vi "MAIN SINUS PENTA.vi"(8 "err in":errorcluster, 10 "SIMULAZIONE":bool=TRUE) -> ()   [LabVIEW 2019]
uses:
  controls/Parametri inverter letti.ctl
  controls/Dati targa sinus penta.ctl
  <vilib>/Utility/file.llb/Read Delimited Spreadsheet (string).vi
  Global dati targa SINUSPENTA.vi
  <vilib>/Modbus/master/Create Master Instance (Serial).vi
  <vilib>/Modbus/master/Modbus Master.lvclass
panel:
  out "register values":u16[](array[numeric])
  in  "modalità stop":i16
  in  "set modalità stop":bool
  out "error out":errorcluster
  out "appended array 3":u16[](array[numeric])
  out "appended array 2":dbl[](array[numeric])
  in  "DATI TARGA sinus penta 2":T1 {"Potenza nominale del motore Mot1" format="%.1f"; "Corrente nominale del motore Mot1" format="%.1f"; "Tensione nominale del motore mot1" format="%.1f"}
  out "# elements in queue":i32
  in  "START ABILITA":bool
  out "data 2":dbl
  out "Freq nominale del motore Mot1":u16
  out "DATI TARGA sinus penta":T1
  out "appended array":u16[](array[numeric])
  out "RPM nominali del motore Mot1":u16
  in  "set dati targa":bool
  in  "set rampa":bool
  in  "rampa":dbl
  in  "connetti":bool
  in  "disconnetti":bool
  out "data":dbl
  in  "Abilitato":bool
  in  "in marcia":bool=TRUE
  in  "SETUP PORTA SERIALE":T2={"Porta COM"="COM8", "Baud Rate"=38400, "Parity"=0, "Flow Control"=0, "Timeout"=10000, "Mode"=enum."RTU", "Slave Address"=1} {"Flow Control" items=["None", "XON/XOFF", "RTS/CTS", "XON/XOFF & RTS/CTS", "DTR/DSR", "XON/XOFF & DTR/DSR"]; "Parity" items=["None", "Odd", "Even", "Mark", "Space"]}
  out "t":errorcluster
  in  "Visualizza numero registri":bool
  in  "stop":bool
  in  "holding register values":i16[](array[numeric])
  in  "starting address":u16
  in  "write register":bool
  out "READ SINUS PENTA":T3
  out "Numeric":i32
  out "STATO":string
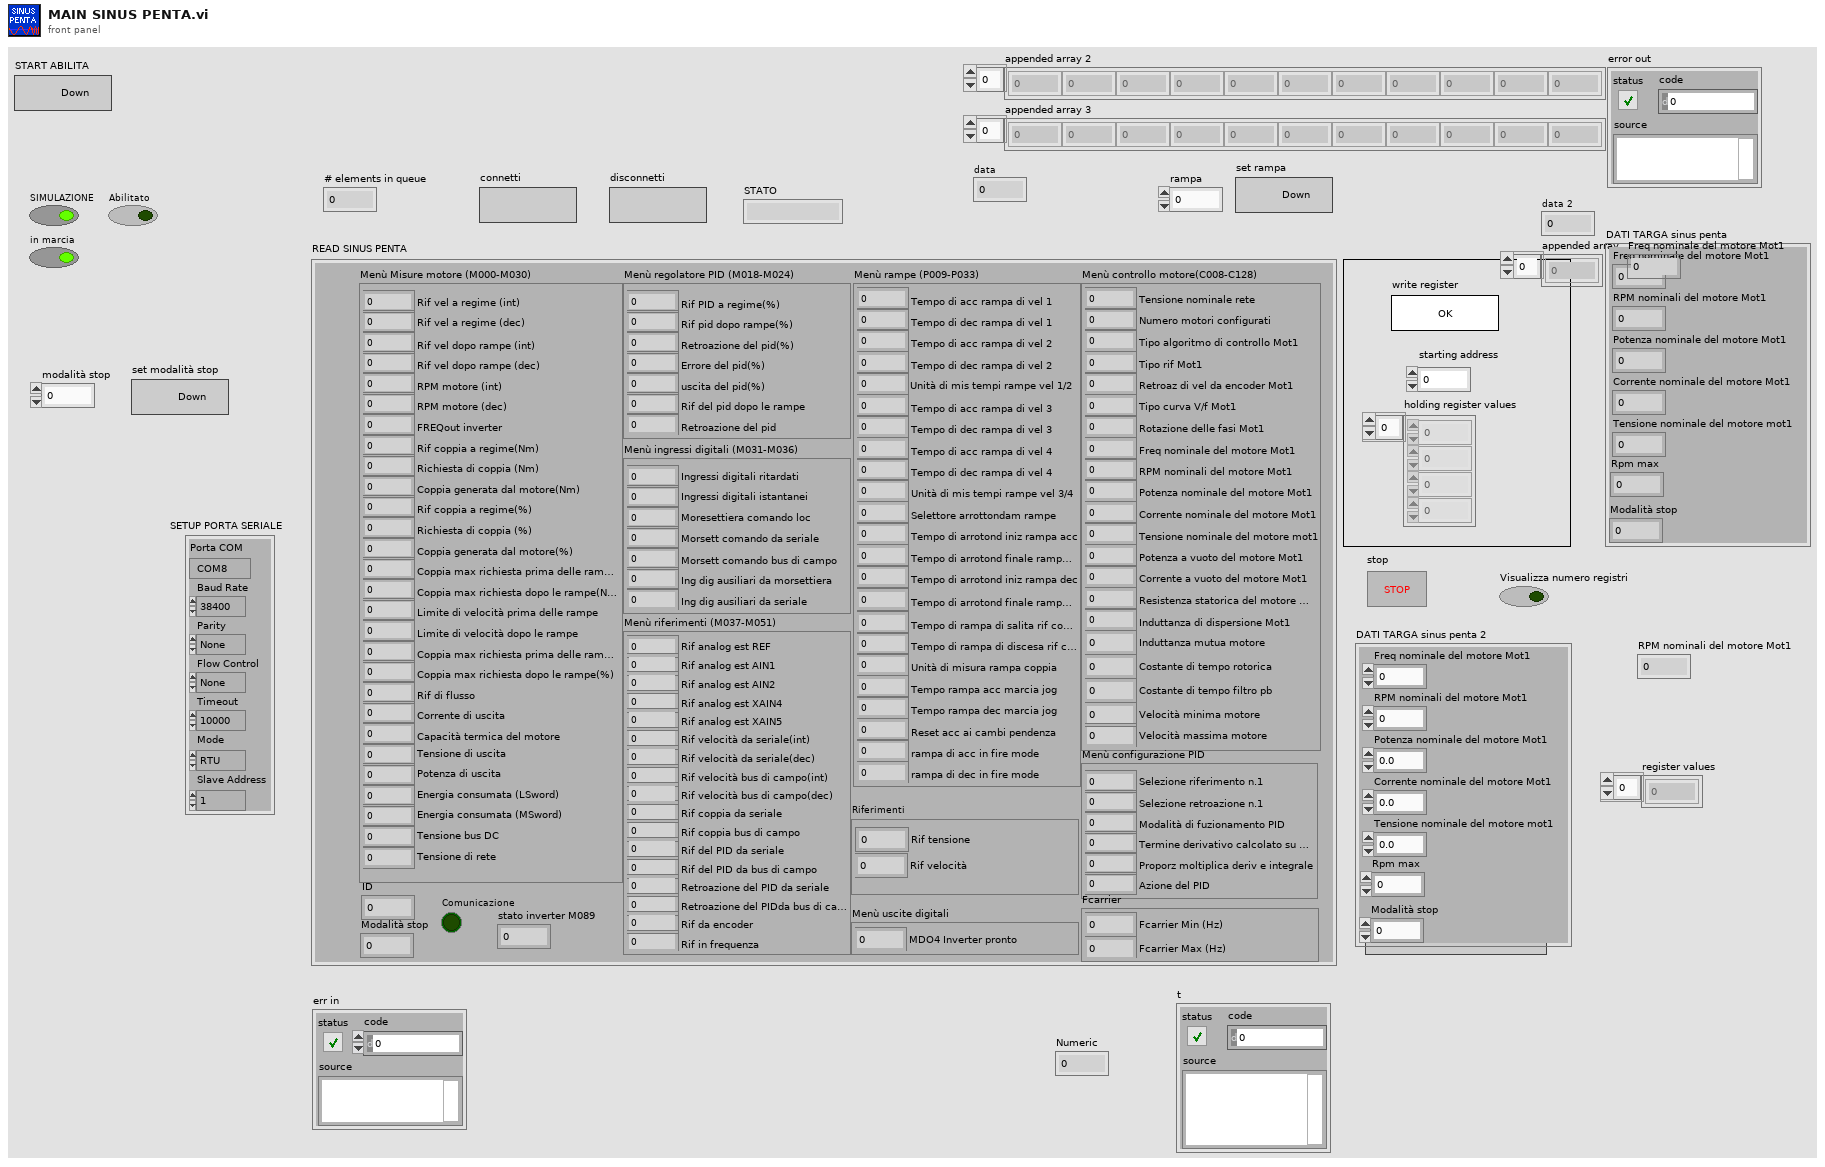
[diagram p1: front panel]
types:
  T1 = typedef "Dati targa sinus penta.ctl" = cluster{"Freq nominale del motore Mot1":dbl, "RPM nominali del motore Mot1":i16, "Potenza nominale del motore Mot1":dbl, "Corrente nominale del motore Mot1":dbl, "Tensione nominale del motore mot1":dbl, "Rpm max":u16, "Modalità stop":u16}
  T2 = cluster{"Porta COM":string, "Baud Rate":u32, "Parity":u16, "Flow Control":u16, "Timeout":u32, "Mode":enum16{"RTU", "ASCII"}, "Slave Address":u8}
  T3 = typedef "Parametri inverter letti.ctl" = cluster{"Menù Misure motore (M000-M030)":cluster{"Rif vel a regime (int)":u16, "Rif vel a regime (dec)":u16, "Rif vel dopo rampe (int)":u16, "Rif vel dopo rampe (dec)":u16, "RPM motore (int)":u16, "RPM motore (dec)":u16, "FREQout inverter":u16, "Rif coppia a regime(Nm)":u16, "Richiesta di coppia (Nm)":u16, "Coppia generata dal motore(Nm)":u16, "Rif coppia a regime(%)":u16, "Richiesta di coppia (%)":u16, "Coppia generata dal motore(%)":u16, "Coppia max richiesta prima delle rampe(Nm)":u16, "Coppia max richiesta dopo le rampe(Nm)":u16, "Limite di velocità prima delle rampe":u16, "Limite di velocità dopo le rampe":u16, "Coppia max richiesta prima delle rampe(%)":u16, "Coppia max richiesta dopo le rampe(%)":u16, "Rif di flusso":u16, "Corrente di uscita":u16, "Capacità termica del motore":u16, "Tensione di uscita":u16, "Potenza di uscita":u16, "Energia consumata (LSword)":u16, "Energia consumata (MSword)":u16, "Tensione bus DC":u16, "Tensione di rete":u16}, "Menù regolatore PID (M018-M024)":cluster{"Rif PID a regime(%)":u16, "Rif pid dopo rampe(%)":u16, "Retroazione del pid(%)":u16, "Errore del pid(%)":u16, "uscita del pid(%)":u16, "Rif del pid dopo le rampe":u16, "Retroazione del pid":u16}, "Menù ingressi digitali (M031-M036)":cluster{"Ingressi digitali ritardati":u16, "Ingressi digitali istantanei":u16, "Moresettiera comando loc":u16, "Morsett comando da seriale":u16, "Morsett comando bus di campo":u16, "Ing dig ausiliari da morsettiera":u16, "Ing dig ausiliari da seriale":u16}, "Menù riferimenti (M037-M051)":cluster{"Rif analog est REF":u16, "Rif analog est AIN1":u16, "Rif analog est AIN2":u16, "Rif analog est XAIN4":u16, "Rif analog est XAIN5":u16, "Rif velocità da seriale(int)":u16, "Rif velocità bus di campo(int)":u16, "Rif coppia da seriale":u16, "Rif coppia bus di campo":u16, "Rif del PID da seriale":u16, "Rif del PID da bus di campo":u16, "Retroazione del PID da seriale":u16, "Retroazione del PIDda bus di campo":u16, "Rif da encoder":u16, "Rif in frequenza":u16, "Rif velocità da seriale(dec)":u16, "Rif velocità bus di campo(dec)":u16}, "Menù rampe (P009-P033)":cluster{"Tempo di dec rampa di vel 1":u16, "Tempo di acc rampa di vel 2":u16, "Tempo di dec rampa di vel 2":u16, "Tempo di acc rampa di vel 1":u16, "Unità di mis tempi rampe vel 1/2":u16, "Tempo di acc rampa di vel 3":u16, "Tempo di dec rampa di vel 3":u16, "Tempo di acc rampa di vel 4":u16, "Tempo di dec rampa di vel 4":u16, "Unità di mis tempi rampe vel 3/4":u16, "Selettore arrottondam rampe":u16, "Tempo di arrotond iniz rampa acc":u16, "Tempo di arrotond finale rampa acc":u16, "Tempo di arrotond iniz rampa dec":u16, "Tempo di rampa di salita rif coppia":u16, "Tempo di rampa di discesa rif coppia":u16, "Unità di misura rampa coppia":u16, "Tempo rampa acc marcia jog":u16, "Tempo rampa dec marcia jog":u16, "Reset acc ai cambi pendenza":u16, "rampa di acc in fire mode":u16, "rampa di dec in fire mode":u16, "Tempo di arrotond finale rampa dec":u16}, "Menù controllo motore(C008-C128)":cluster{"Numero motori configurati":u16, "Tipo algoritmo di controllo Mot1":u16, "Tipo rif Mot1":u16, "Tensione nominale rete":u16, "Retroaz di vel da encoder Mot1":u16, "Tipo curva V/f Mot1":u16, "Rotazione delle fasi Mot1":u16, "Freq nominale del motore Mot1":u16, "RPM nominali del motore Mot1":u16, "Potenza nominale del motore Mot1":u16, "Corrente nominale del motore Mot1":u16, "Tensione nominale del motore mot1":u16, "Potenza a vuoto del motore Mot1":u16, "Corrente a vuoto del motore Mot1":u16, "Resistenza statorica del motore Mot1":u16, "Induttanza di dispersione Mot1":u16, "Induttanza mutua motore":u16, "Costante di tempo rotorica":u16, "Costante di tempo filtro pb":u16, "Velocità minima motore":u16, "Velocità massima motore":u16}, "Menù configurazione PID":cluster{"Selezione riferimento n.1":u16, "Selezione retroazione n.1":u16, "Modalità di fuzionamento PID":u16, "Termine derivativo calcolato su err o mis":u16, "Proporz moltiplica deriv e integrale":u16, "Azione del PID":u16}, "ID":dbl, "Menù uscite digitali":cluster{"MDO4 Inverter pronto":u16}, "Fcarrier":cluster{"Fcarrier Min (Hz)":u16, "Fcarrier Max (Hz)":u16}, "stato inverter M089":dbl, "Riferimenti":cluster{"Rif tensione":u16, "Rif velocità":u16}, "Comunicazione":bool, "Modalità stop":dbl}
  T4 = cluster{"Array of elements":cluster{"String":string, "variant":variant}[], "Single element":cluster{"String":string, "variant":variant}, "enque at\nopposite end (F)":bool, "no replications (F)":bool}
  T5 = cluster{"Trampa[s] acc":dbl, "Trampa[s] dec":dbl}
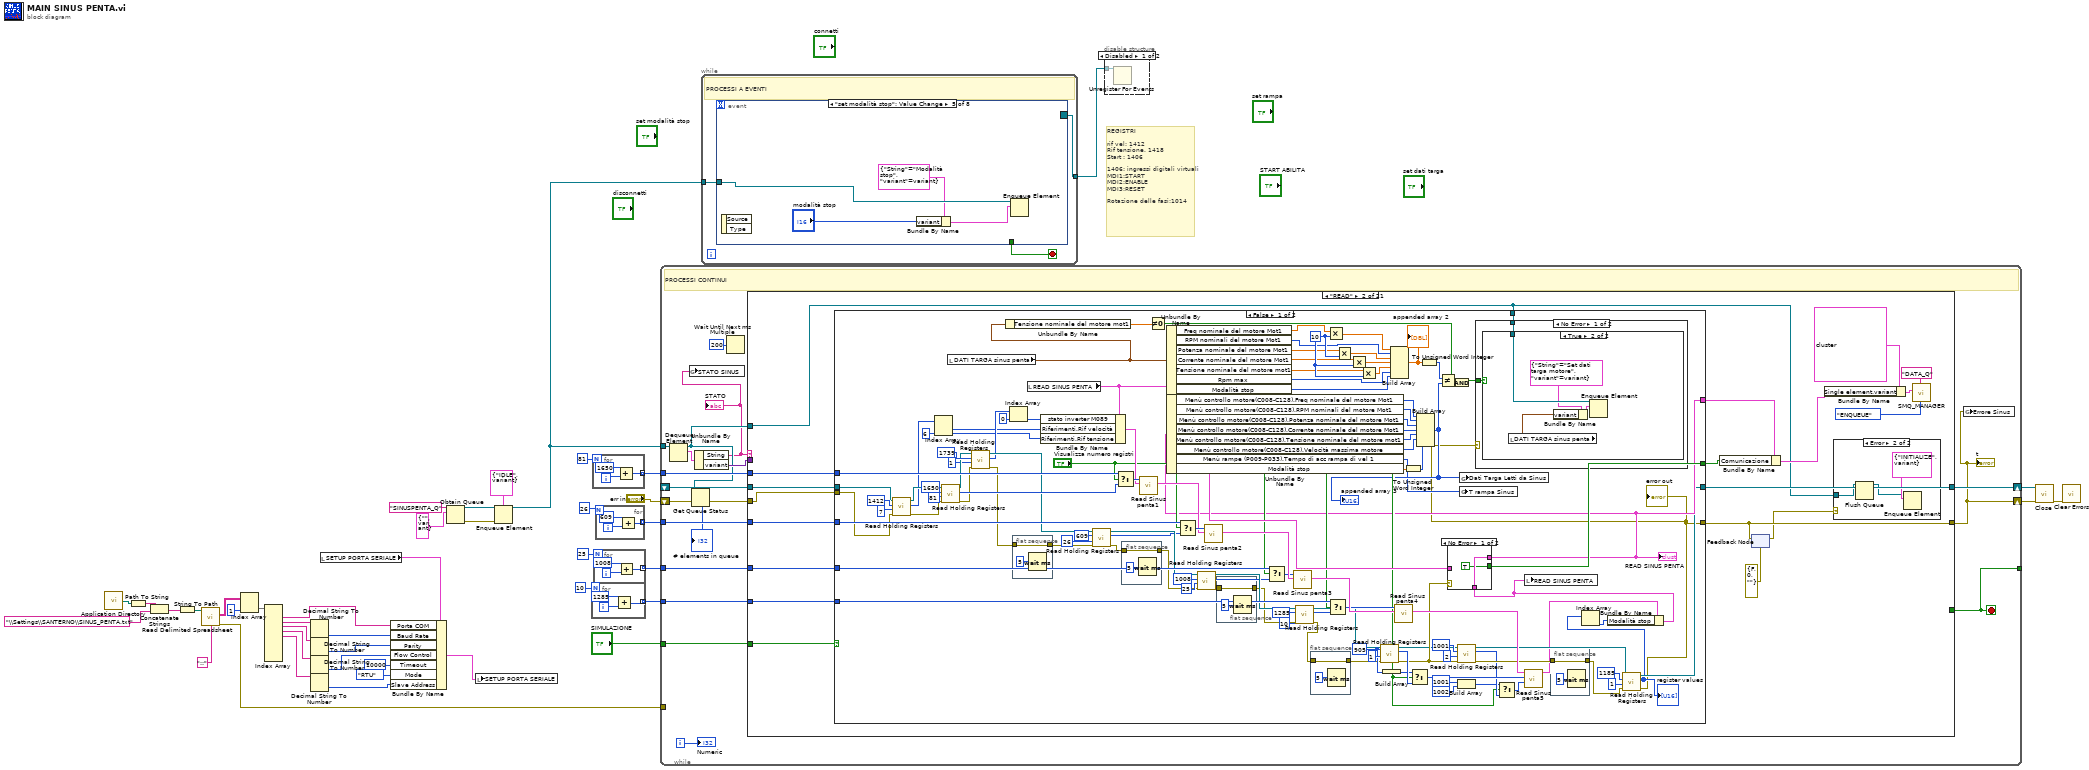
[diagram p0: block diagram]
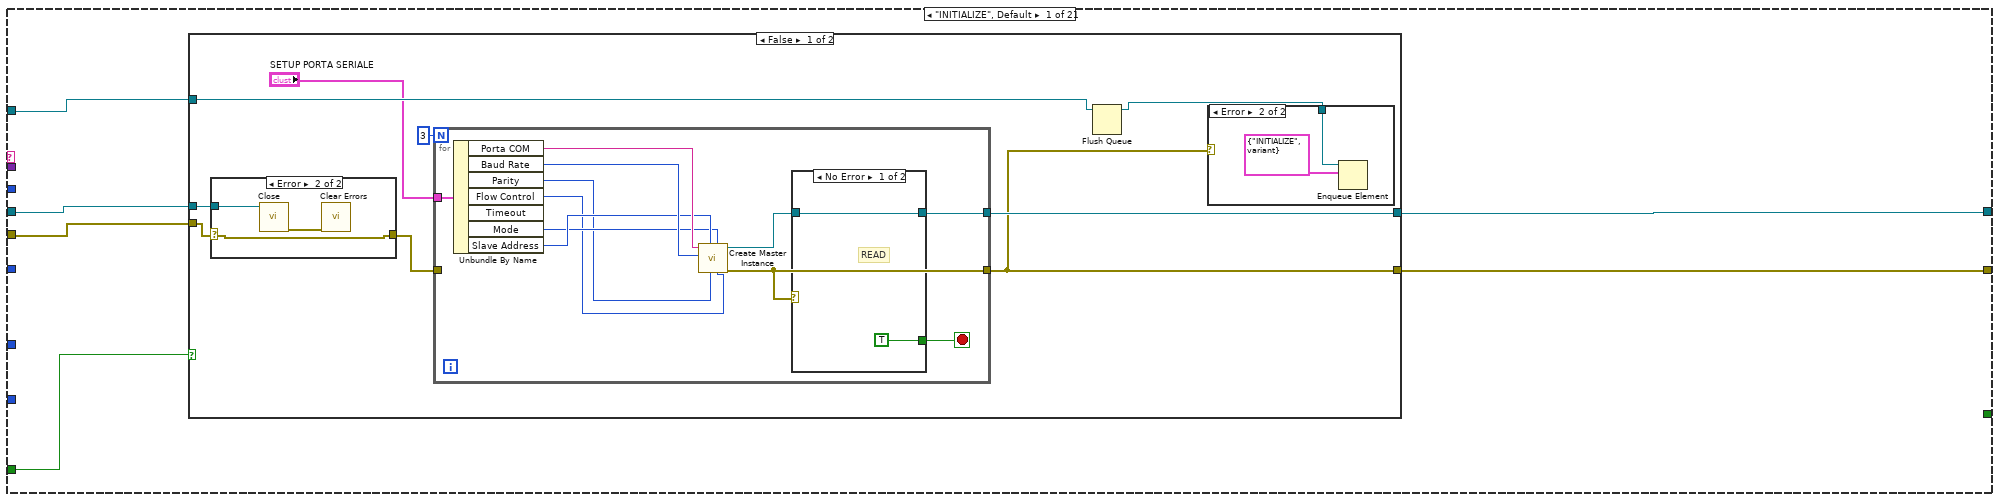
[diagram p3: hidden frame]
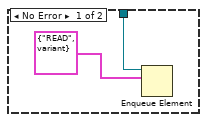
[diagram p4: hidden frame]
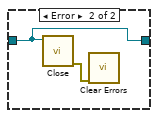
[diagram p6: hidden frame]
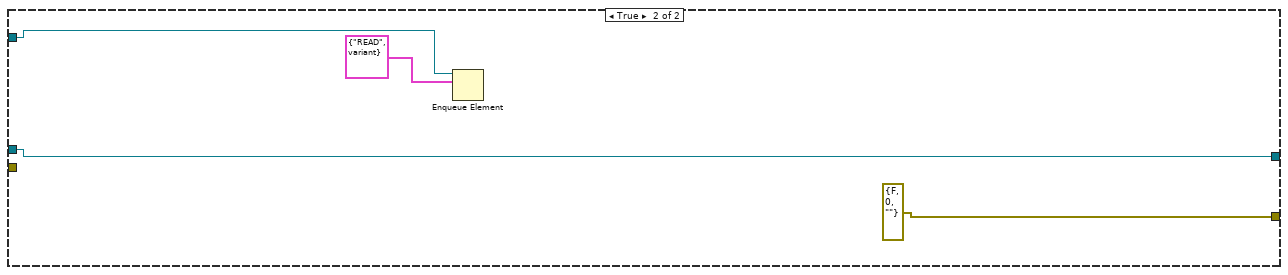
[diagram p7: hidden frame]
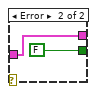
[diagram p10: hidden frame]
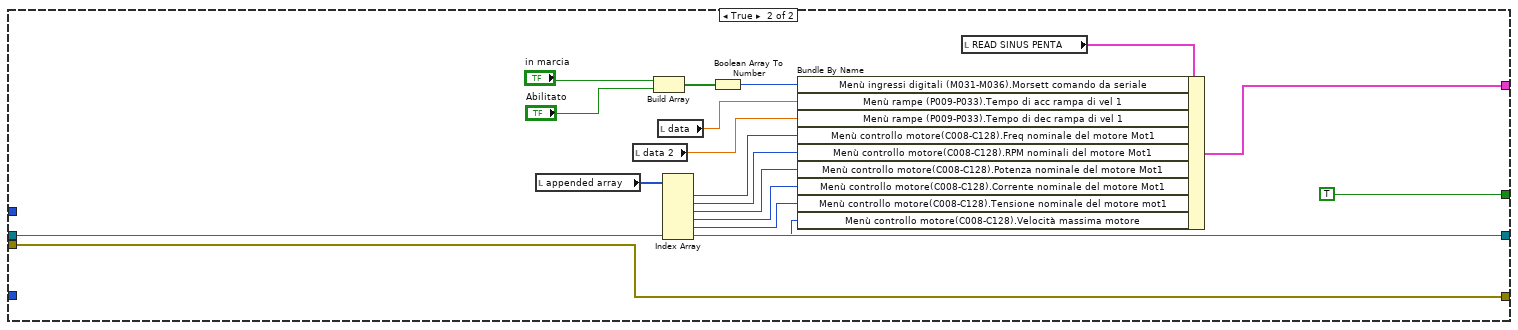
[diagram p11: hidden frame]
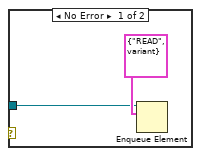
[diagram p12: hidden frame]
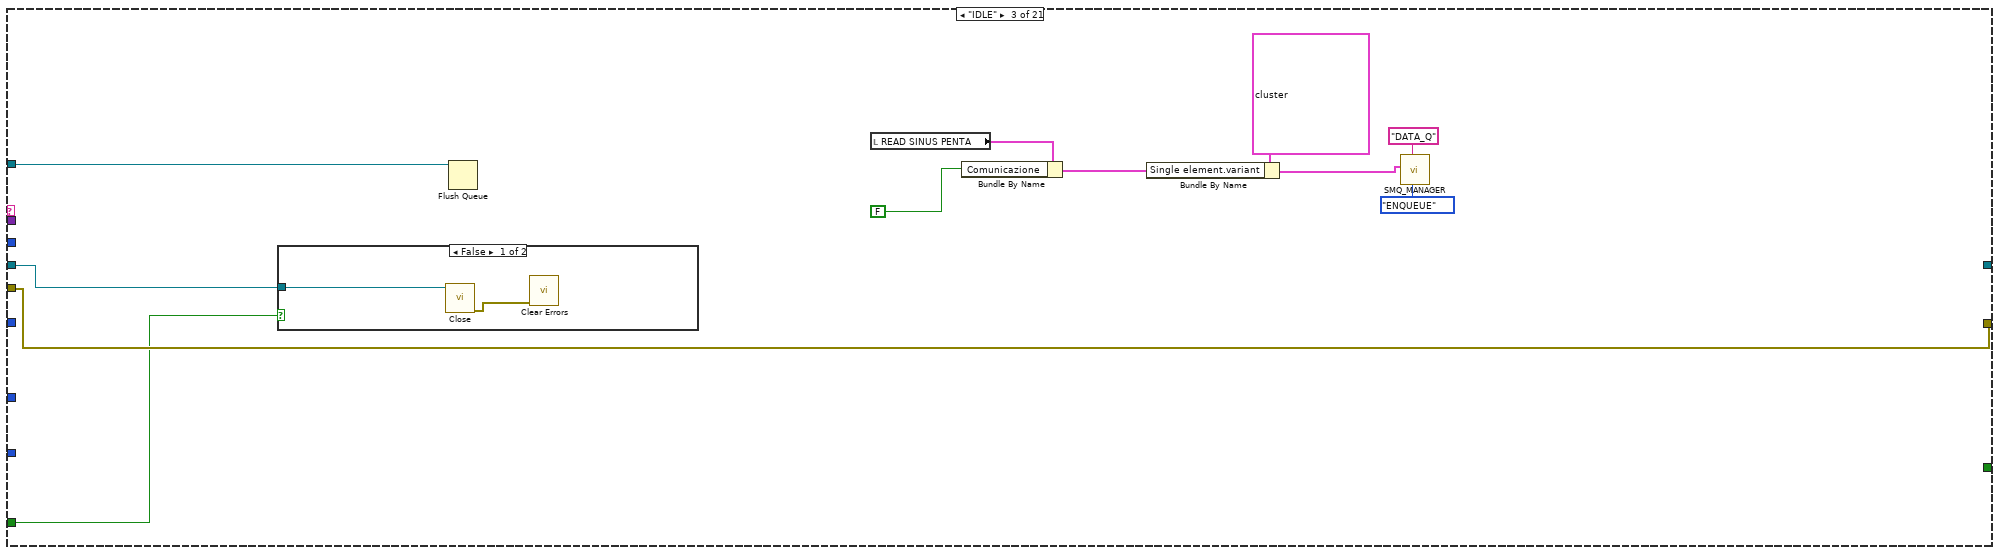
[diagram p13: hidden frame]
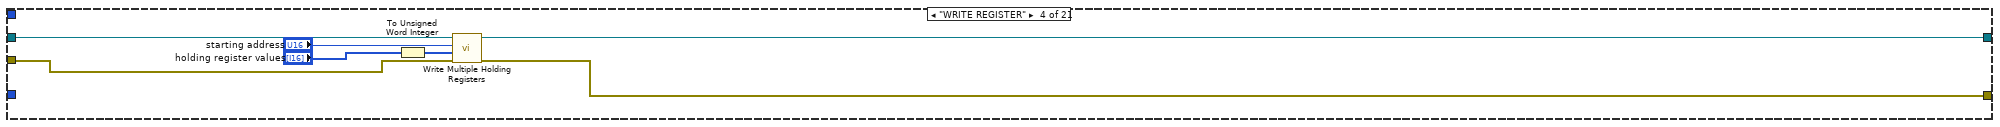
[diagram p15: hidden frame]
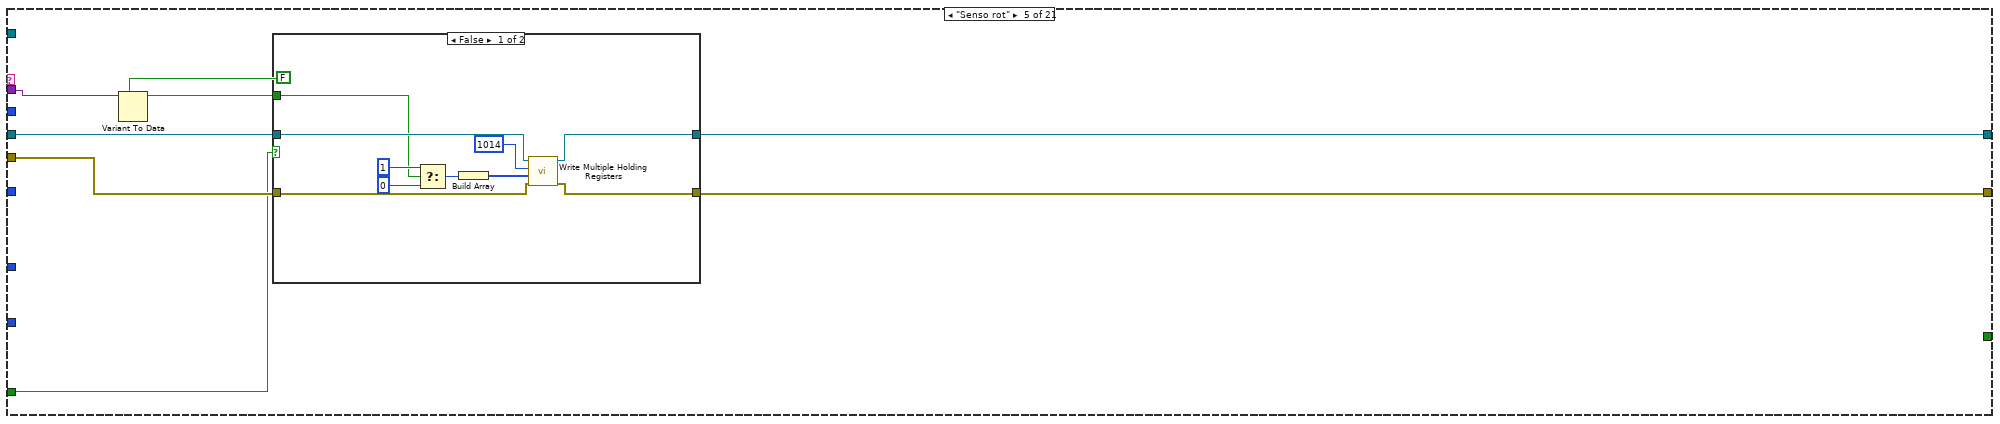
[diagram p16: hidden frame]
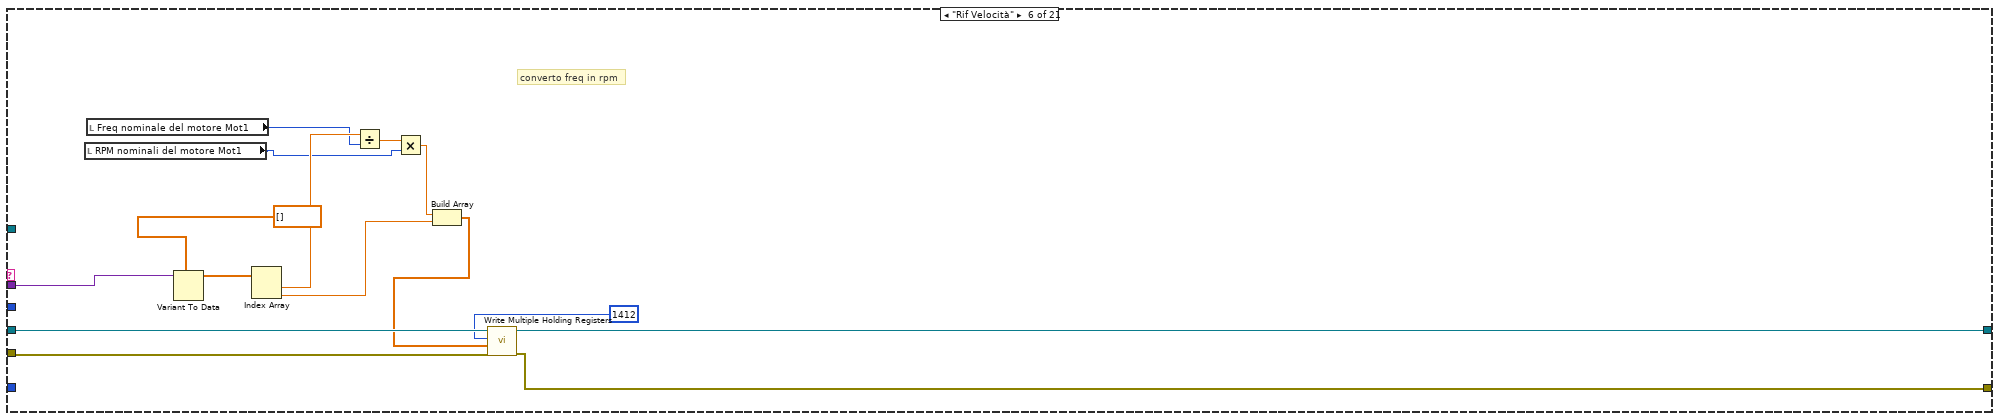
[diagram p18: hidden frame]
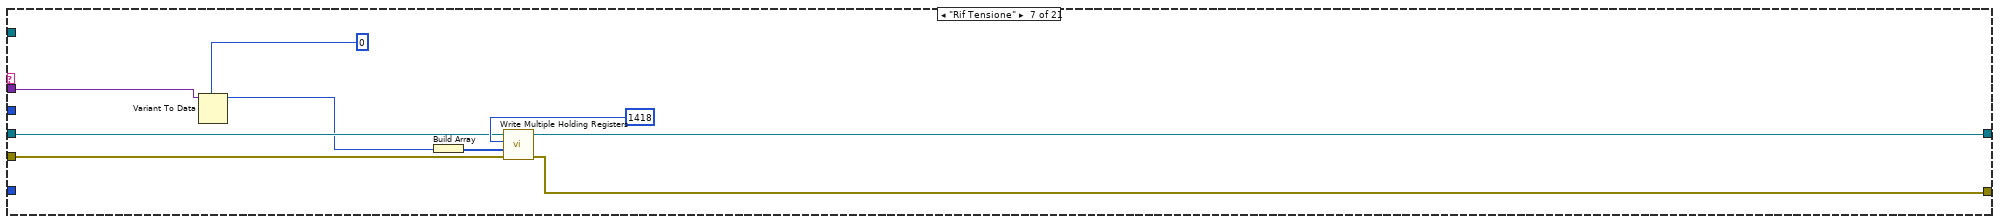
[diagram p19: hidden frame]
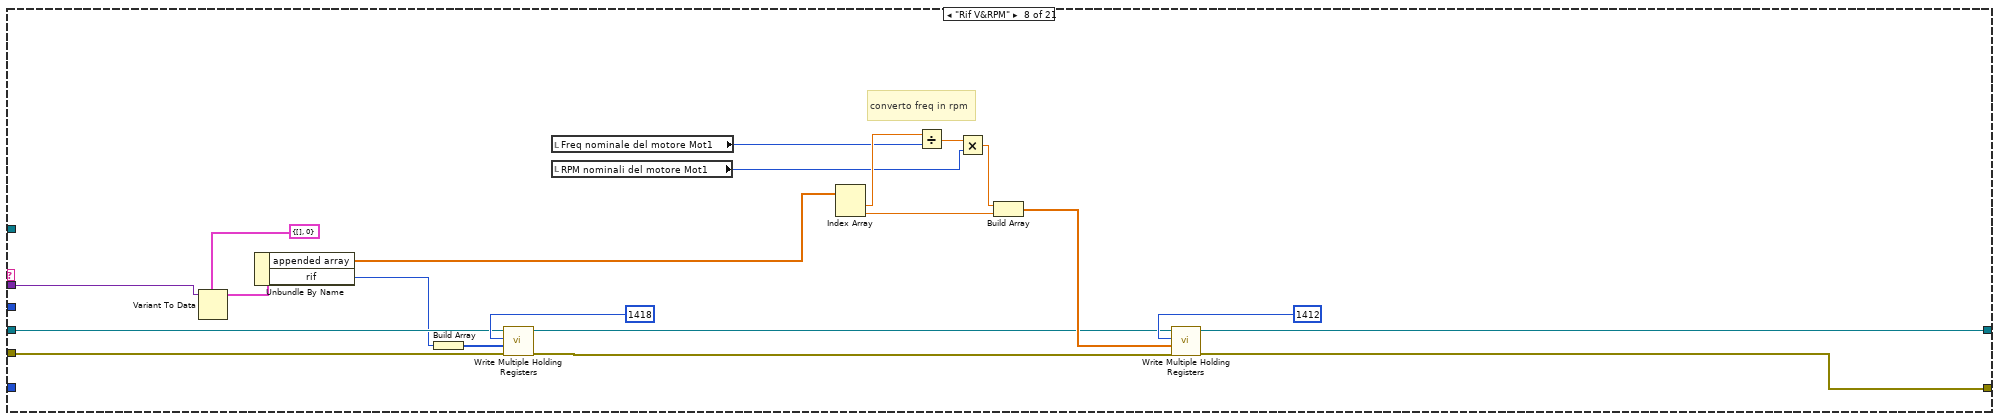
[diagram p20: hidden frame]
diagram:
  # "REGISTRI\n\nrif vel: 1412\nRif tensione. 1418\nStart : 1406\n\n1406: ingressi digitali virtuali\nMDI1:START\nMDI2:ENABLE\nMDI3:RESET\n\nRotazione delle fasi:1014"
  n1 = call <vilib>:"Application Directory.vi"() -> ("Application Directory"=w12:path)
  n2 = Path To String(path=w12) -> (string=w13:string)
  n3 = Concatenate Strings(w13, "\\Settings\\SANTERNO\\SINUS_PENTA.txt" ("string")) -> (w15:string)
  n4 = String To Path(string=w15) -> (path=w16:path)
  n5 = call-poly <vilib>:"Read Delimited Spreadsheet.vi"("file path (dialog if empty)"=w16, "delimiter (\\t)"="::" ("delimiter (\\t)")) -> ("all rows"=w17:string[][], "error out"=w2:errorcluster)  [unwired: 8 in, 4 out]
  n6 = Index Array(array=w17, index (col)=1 ("disabled index (col)")) -> (element=w19:string[])  [unwired: 1 in]
  n7 = Index Array(array=w19) -> (element #1=w10:string, element #2=w20:string, element #3=w21:string, element #4=w22:string, element #5=w23:string)  [unwired: 10 in, 5 out]
  n8 = Decimal String To Number(string=w20) -> (number=w9:i32)  [unwired: 2 in, 1 out]
  n9 = Decimal String To Number(string=w21) -> (number=w8:i32)  [unwired: 2 in, 1 out]
  n10 = Decimal String To Number(string=w22) -> (number=w7:i32)  [unwired: 2 in, 1 out]
  n11 = Decimal String To Number(string=w23) -> (number=w5:i32)  [unwired: 2 in, 1 out]
  n12 = local read "SETUP PORTA SERIALE"() -> (w4:T2)
  n13 = Bundle By Name(cluster=w4, "Porta COM"=w10, "Baud Rate"=w9, "Parity"=w8, "Flow Control"=w7, "Timeout"=u32 10000, "Mode"=enum16{"RTU", "ASCII"}."RTU", "Slave Address"=w5) -> (w3:T2)
  n14 = Obtain Queue(name (unnamed)="SINUSPENTA_Q", element data type=cluster{"String":string, "variant":variant} {"String"="", "variant"=variant} ("element")) -> (queue out=w25:refnum<queue>, error out=w27:errorcluster)  [unwired: 3 in, 1 out]
  n15 = local write "SETUP PORTA SERIALE"(w3) -> ()
  n16 = Enqueue Element(queue=w25, element=cluster{"String":string, "variant":variant} {"String"="IDLE", "variant"=variant}, error in (no error)=w27) -> (queue out=w43:refnum<queue>)  [unwired: 1 in, 2 out]
  n17 = for {
    N: 10 -> [_]
    tunnel: [w44] -> w35 mode=indexing
    i -> [w46]
    n18 = Add(x=1285, y=w46) -> (x+y=w44:i32)
  }
  n19 = for {
    N: 81 -> [_]
    tunnel: [w47] -> w41 mode=indexing
    i -> [w49]
    n20 = Add(x=1650, y=w49) -> (x+y=w47:i32)
  }
  n21 = for {
    N: 25 -> [_]
    tunnel: [w50] -> w37 mode=indexing
    i -> [w52]
    n22 = Add(x=1008, y=w52) -> (x+y=w50:i32)
  }
  n23 = for {
    N: 26 -> [_]
    tunnel: [w53] -> w39 mode=indexing
    i -> [w55]
    n24 = Add(x=609, y=w55) -> (x+y=w53:i32)
  }
  n25 = while {
    shift-right: [w57] -> w33
    shift-left: "err in" -> [w73]
    tunnel: w43 -> [w64]
    tunnel: [w61] -> _
    shift-right: [w65] -> w34
    shift-left: _ -> [w70]
    tunnel: w41 -> [w69]
    tunnel: w39 -> [w68]
    tunnel: w37 -> [w67]
    tunnel: w35 -> [w66]
    tunnel: "SIMULAZIONE" -> [w60]
    tunnel: w2 -> [_]
    i -> [w71]
    stop <- w61 stop-if-true
    # "PROCESSI CONTINUI"
    n26 = Dequeue Element(queue=w64) -> (queue out=w59:refnum<queue>, element=w63:cluster{"String":string, "variant":variant})  [unwired: 2 in, 2 out]
    n27 = Get Queue Status(queue=w59) -> (# elements in queue=→"# elements in queue":i32)  [unwired: 2 in, 7 out]
    n28 = Unbundle By Name(w63) -> ("String"=w56:string, "variant"=w62:variant)
    "STATO" <- w56
    n29 = global write "Global dati targa SINUSPENTA.vi" "STATO SINUS"(w56) -> ()
    n30 = Wait Until Next ms Multiple(millisecond multiple=u32 200 ("milliseconds to wait")) -> ()  [unwired: 1 out]
    n31 = case shown="\"READ\"" w56 {
      tunnel: [_ _ _ _ _ _ _ _ _ _ _ _ _ _ _ _ _ _ _ _ TRUE] -> w61
      tunnel: w73 -> [w77 w128 w301 w306 w317 w343 w353 w374 w383 w390 w404 w415 w427 w460 w502 w506 w513 w525 w546 w576 w604]
      tunnel: [w75 w118 w301 w305 w316 w342 w349 w358 w382 w393 w403 w414 w426 w459 w495 w506 w510 w523 w544 w559 w604] -> w57
      tunnel: w62 -> [_ _ _ _ w314 w340 w350 w372 _ _ _ _ _ _ w500 _ _ w522 w543 w583 _]
      tunnel: w59 -> [w79 w119 w300 _ _ _ _ _ w378 w388 w401 w412 _ _ _ _ _ _ _ _ _]
      tunnel: [w76 w130 _ w307 w315 w344 w351 w360 w380 w391 w405 w416 w424 w461 w493 w505 w511 w524 w545 w558 w603] -> w65
      tunnel: w70 -> [w78 w129 w299 w310 w318 w345 w352 w373 w381 w392 w406 w417 w425 w462 w501 w505 w512 w526 w547 w577 w603]
      tunnel: w69 -> [_ w134 _ _ _ _ _ _ _ _ _ _ _ _ _ _ _ _ _ _ _]
      tunnel: w68 -> [_ w133 _ _ _ _ _ _ _ _ _ _ _ _ _ _ _ _ _ _ _]
      tunnel: w67 -> [_ w132 _ _ _ _ _ _ _ _ _ _ _ _ _ _ _ _ _ _ _]
      tunnel: w66 -> [_ w131 _ _ _ _ _ _ _ _ _ _ _ _ _ _ _ _ _ _ _]
      tunnel: w60 -> [w74 w127 w298 _ w311 _ _ _ _ _ _ _ _ _ _ _ _ w521 w542 w572 _]
      frame "INITIALIZE", Default {
        n32 = case shown="False" w74 {
          tunnel: [w87 w115] -> w76
          tunnel: w78 -> [w86 w115]
          tunnel: w79 -> [w82 w113]
          tunnel: [w84 errorcluster {"status"=FALSE, "code"=0, "source"=""} ("err in 2")] -> w75
          tunnel: w77 -> [w83 _]
          frame False {
            n33 = case shown="Error" w83 {
              selector: w83 -> [w93 w95]
              tunnel: w86 -> [_ w96]
              tunnel: [w93 w95] -> w85
              frame No Error {
              }
              frame Error {
                n34 = call-dynamic "Close.vi"("Modbus master in"=w96) -> ("error out"=w94:errorcluster)  [unwired: 10 in]
                n35 = call <vilib>:"Clear Errors.vi"("error in (no error)"=w94) -> ()  [unwired: 5 in, 2 out]
              }
            }
            n36 = for {
              N: 3 -> [_]
              tunnel: w85 -> [_]
              tunnel: "SETUP PORTA SERIALE" -> [w107]
              tunnel: [w100] -> w84
              tunnel: [w98] -> w87
              stop <- w97 stop-if-true
              n37 = Unbundle By Name(w107) -> ("Porta COM"=w106:string, "Baud Rate"=w105:u32, "Parity"=w102:u16, "Flow Control"=w101:u16, "Mode"=w103:enum16{"RTU", "ASCII"}, "Slave Address"=w104:u8)  [unwired: 1 out]
              n38 = call-poly <vilib>:"Create Master Instance.vi"("flow control (None)"=w101, "serial type"=w103, "parity (Even)"=w102, "unit ID"=w104, "baud rate (9600)"=w105, "VISA resource name"=w106) -> ("error out"=w100:errorcluster, "serial master instance"=w99:refnum<class "Modbus Master.lvclass">)  [unwired: 4 in]
              n39 = case shown="No Error" w100 {
                tunnel: w99 -> [w109 w111]
                tunnel: [w109 w111] -> w98
                tunnel: [TRUE _] -> w97
                frame No Error {
                  # "READ"
                }
                frame Error {
                  n40 = call-dynamic "Close.vi"("Modbus master in"=w111) -> ("error out"=w110:errorcluster)  [unwired: 10 in]
                  n41 = call <vilib>:"Clear Errors.vi"("error in (no error)"=w110) -> ()  [unwired: 5 in, 2 out]
                }
              }
            }
            n42 = Flush Queue(queue=w82) -> (queue out=w81:refnum<queue>)  [unwired: 1 in, 2 out]
            n43 = case shown="Error" w84 {
              tunnel: w81 -> [w89 w91]
              frame No Error {
                n44 = Enqueue Element(queue=w89, element=cluster{"String":string, "variant":variant} {"String"="READ", "variant"=variant}) -> ()  [unwired: 2 in, 3 out]
              }
              frame Error {
                n45 = Enqueue Element(queue=w91, element=cluster{"String":string, "variant":variant} {"String"="INITIALIZE", "variant"=variant}) -> ()  [unwired: 2 in, 3 out]
              }
            }
          }
          frame True {
            n46 = Enqueue Element(queue=w113, element=cluster{"String":string, "variant":variant} {"String"="READ", "variant"=variant}) -> ()  [unwired: 2 in, 3 out]
          }
        }
      }
      frame "READ" {
        n47 = case shown="False" w127 {
          tunnel: w134 -> [w247 _]
          tunnel: w133 -> [w246 _]
          tunnel: w132 -> [w245 _]
          tunnel: w131 -> [w244 _]
          tunnel: [w144 w285] -> w130
          tunnel: [w135 w284] -> w118
          tunnel: w129 -> [w178 w285]
          tunnel: w128 -> [w177 w284]
          tunnel: [w159 w282] -> w122
          tunnel: [w176 TRUE ("Visualizza numero registri")] -> w120
          tunnel: w119 -> [w157 _]
          frame False {
            w171 = u16 10 ("y")
            w217 = u16 905 ("starting address")
            n48 = call-dynamic "Read Holding Registers.vi"("error in (no error)"=w177, "number of holding registers"=u16 7, "starting address"=u16 1412, "Modbus master in"=w178) -> ("error out"=w185:errorcluster, "register values"=w182:u16[], "Modbus master out"=w186:refnum<class "Modbus Master.lvclass">)  [unwired: 5 in]
            n49 = Index Array(array=w182, index #2=6 ("index")) -> (element #1=w180:u16, element #2=w179:u16)  [unwired: 1 in]
            n50 = call-dynamic "Read Holding Registers.vi"("error in (no error)"=w185, "number of holding registers"=u16 81, "starting address"=u16 1650, "Modbus master in"=w186) -> ("error out"=w184:errorcluster, "register values"=w225:u16[], "Modbus master out"=w194:refnum<class "Modbus Master.lvclass">)  [unwired: 5 in]
            n51 = local read "DATI TARGA sinus penta"() -> (w155:T1)
            n52 = call-dynamic "Read Holding Registers.vi"("error in (no error)"=w184, "number of holding registers"=u16 1, "starting address"=u16 1739, "Modbus master in"=w194) -> ("error out"=w183:errorcluster, "register values"=w191:u16[], "Modbus master out"=w193:refnum<class "Modbus Master.lvclass">)  [unwired: 5 in]
            n53 = Unbundle By Name(w155) -> ("Tensione nominale del motore mot1"=w154:dbl)
            n54 = Index Array(array=w191, index=0) -> (element=w189:u16)
            n55 = flat-sequence {
              tunnel: w183 -> [w262]
              tunnel: [w262] -> w213
              frame #0 {
                n56 = Wait (ms)(milliseconds to wait=u32 5) -> ()  [unwired: 1 out]
              }
            }
            n57 = local read "READ SINUS PENTA"() -> (w214:T3)
            n58 = Bundle By Name(cluster=w214, "stato inverter M089"=w189, "Riferimenti.Rif velocità"=w180, "Riferimenti.Rif tensione"=w179) -> (w223:T3)
            n59 = call-dynamic "Read Holding Registers.vi"("error in (no error)"=w213, "number of holding registers"=u16 26, "starting address"=u16 609, "Modbus master in"=w193) -> ("error out"=w212:errorcluster, "register values"=w227:u16[], "Modbus master out"=w239:refnum<class "Modbus Master.lvclass">)  [unwired: 5 in]
            n60 = Select(t=w247, s="Visualizza numero registri", f=w225) -> (s? t:f=w224:i32[])
            n61 = flat-sequence {
              tunnel: w212 -> [w260]
              tunnel: [w260] -> w211
              frame #0 {
                n62 = Wait (ms)(milliseconds to wait=u32 5) -> ()  [unwired: 1 out]
              }
            }
            n63 = call "Read Sinus penta1.vi"("Parametri inverter 2"=w223, "register values"=w224) -> ("output cluster"=w222:T3)  [unwired: 9 in]
            n64 = Not Equal To 0?(x=w154) -> (x != 0?=w153:bool)
            n65 = Unbundle By Name(w155) -> ("Freq nominale del motore Mot1"=w170:dbl, "RPM nominali del motore Mot1"=w169:i16, "Potenza nominale del motore Mot1"=w168:dbl, "Corrente nominale del motore Mot1"=w167:dbl, "Tensione nominale del motore mot1"=w166:dbl, "Rpm max"=w150:u16, "Modalità stop"=w139:u16)
            n66 = Select(t=w246, s="Visualizza numero registri", f=w227) -> (s? t:f=w226:i32[])
            n67 = call-dynamic "Read Holding Registers.vi"("error in (no error)"=w211, "number of holding registers"=u16 25, "starting address"=u16 1008, "Modbus master in"=w239) -> ("error out"=w210:errorcluster, "register values"=w229:u16[], "Modbus master out"=w235:refnum<class "Modbus Master.lvclass">)  [unwired: 5 in]
            n68 = call "Read Sinus penta2.vi"("Parametri inverter"=w222, "register values"=w226) -> ("output cluster"=w240:T3)  [unwired: 9 in]
            n69 = flat-sequence {
              tunnel: w210 -> [w258]
              tunnel: [w258] -> w209
              frame #0 {
                n70 = Wait (ms)(milliseconds to wait=u32 5) -> ()  [unwired: 1 out]
              }
            }
            n71 = Select(t=w245, s="Visualizza numero registri", f=w229) -> (s? t:f=w228:i32[])
            n72 = call "Read Sinus penta3.vi"("Parametri inverter"=w240, "register values"=w228) -> ("output cluster"=w234:T3)  [unwired: 9 in]
            n73 = call-dynamic "Read Holding Registers.vi"("error in (no error)"=w209, "number of holding registers"=u16 10, "starting address"=u16 1285, "Modbus master in"=w235) -> ("error out"=w208:errorcluster, "register values"=w231:u16[], "Modbus master out"=w221:refnum<class "Modbus Master.lvclass">)  [unwired: 5 in]
            n74 = flat-sequence {
              tunnel: w208 -> [w256]
              tunnel: [w256] -> w207
              frame #0 {
                n75 = Wait (ms)(milliseconds to wait=u32 5) -> ()  [unwired: 1 out]
              }
            }
            n76 = Multiply(x=w170, y=w171) -> (x*y=w175:dbl)
            n77 = Select(t=w244, s="Visualizza numero registri", f=w231) -> (s? t:f=w230:i32[])
            n78 = Multiply(x=w168, y=w171) -> (x*y=w174:dbl)
            n79 = Multiply(x=w167, y=w171) -> (x*y=w173:dbl)
            n80 = Multiply(x=w166, y=w171) -> (x*y=w172:dbl)
            n81 = call-dynamic "Read Holding Registers.vi"("error in (no error)"=w207, "number of holding registers"=u16 1, "starting address"=w217, "Modbus master in"=w221) -> ("error out"=w205:errorcluster, "register values"=w219:u16[], "Modbus master out"=w196:refnum<class "Modbus Master.lvclass">)  [unwired: 5 in]
            n82 = Build Array(w217) -> (w216:u16[])
            n83 = Build Array(w175, w169, w174, w173, w172, w150, w139) -> (w160:dbl[])
            "appended array 2" <- w160
            n84 = call "Read Sinus penta4.vi"("Parametri inverter"=w234, "register values"=w230) -> ("output cluster"=w215:T3)  [unwired: 9 in]
            n85 = Select(t=w216, s="Visualizza numero registri", f=w219) -> (s? t:f=w218:u16[])
            n86 = To Unsigned Word Integer(number=w160) -> (unsigned 16bit integer=w152:u16[])
            n87 = call-dynamic "Read Holding Registers.vi"("error in (no error)"=w205, "number of holding registers"=u16 2, "starting address"=u16 1001, "Modbus master in"=w196) -> ("error out"=w204:errorcluster, "register values"=w201:u16[], "Modbus master out"=w145:refnum<class "Modbus Master.lvclass">)  [unwired: 5 in]
            n88 = Build Array(u16 1001 ("starting address"), u16 1002 ("element")) -> (w200:u16[])
            n89 = Select(t=w200, s="Visualizza numero registri", f=w201) -> (s? t:f=w202:u16[])
            n90 = call "Read Sinus penta5.vi"("register values 2"=w202, "register values"=w218, "output cluster in"=w215) -> ("output cluster out"=w143:T3)  [unwired: 8 in]
            n91 = flat-sequence {
              tunnel: [w254] -> w136
              tunnel: w204 -> [w254]
              frame #0 {
                n92 = Wait (ms)(milliseconds to wait=u32 5) -> ()  [unwired: 1 out]
              }
            }
            n93 = call-dynamic "Read Holding Registers.vi"("error in (no error)"=w136, "number of holding registers"=u16 1, "starting address"=u16 1185, "Modbus master in"=w145) -> ("error out"=w135:errorcluster, "register values"=w141:u16[], "Modbus master out"=w144:refnum<class "Modbus Master.lvclass">)  [unwired: 5 in]
            "error out" <- w135
            "register values" <- w141
            n94 = Index Array(array=w141) -> (element=w140:u16)  [unwired: 1 in]
            n95 = Bundle By Name(cluster=w143, "Modalità stop"=w140) -> (w142:T3)
            n96 = case shown="No Error" w205 {
              tunnel: w214 -> [_ w267]
              tunnel: [w265 w267] -> w159
              tunnel: w142 -> [w265 _]
              tunnel: [TRUE ("Visualizza numero registri") FALSE ("Visualizza numero registri")] -> w176
              frame No Error {
              }
              frame Error {
              }
            }
            "READ SINUS PENTA" <- w159
            n97 = Unbundle By Name(w159) -> ("Menù controllo motore(C008-C128).Freq nominale del motore Mot1"=w165:u16, "Menù controllo motore(C008-C128).RPM nominali del motore Mot1"=w164:u16, "Menù controllo motore(C008-C128).Potenza nominale del motore Mot1"=w163:u16, "Menù controllo motore(C008-C128).Corrente nominale del motore Mot1"=w162:u16, "Menù controllo motore(C008-C128).Tensione nominale del motore mot1"=w161:u16, "Menù controllo motore(C008-C128).Velocità massima motore"=w149:u16, "Menù rampe (P009-P033).Tempo di acc rampa di vel 1"=w148:u16, "Modalità stop"=w138:dbl)
            n98 = To Unsigned Word Integer(number=w138) -> (unsigned 16bit integer=w137:u16)
            n99 = Build Array(w165, w164, w163, w162, w161, w149, w137) -> (w151:u16[])
            "appended array 3" <- w151
            n100 = Not Equal?(x=w152, y=w151) -> (x != y?=w158:bool)
            n101 = And(x=w158, y=w153) -> (x .and. y?=w156:bool)
            n102 = global write "Global dati targa SINUSPENTA.vi" "T rampa Sinus"(w148) -> ()
            n103 = global write "Global dati targa SINUSPENTA.vi" "Dati Targa Letti da Sinus"(w151) -> ()
            n104 = case shown="No Error" w135 {
              tunnel: w156 -> [w249 _]
              tunnel: w157 -> [w248 _]
              frame No Error {
                n105 = case shown="True" w249 {
                  tunnel: w248 -> [_ w253]
                  frame False {
                  }
                  frame True {
                    n106 = local read "DATI TARGA sinus penta"() -> (w250:T1)
                    n107 = Bundle By Name(cluster=cluster{"String":string, "variant":variant} {"String"="Set dati targa motore", "variant"=variant} ("element"), "variant"=w250) -> (w251:cluster{"String":string, "variant":variant})
                    n108 = Enqueue Element(queue=w253, element=w251) -> ()  [unwired: 2 in, 3 out]
                  }
                }
              }
              frame Error {
              }
            }
            n109 = local write "READ SINUS PENTA"(w142) -> ()
          }
          frame True {
            n110 = local read "appended array"() -> (w274:u16[])
            n111 = local read "data 2"() -> (w275:dbl)
            n112 = Build Array("in marcia", "Abilitato") -> (w279:bool[])
            n113 = local read "data"() -> (w276:dbl)
            n114 = Index Array(array=w274) -> (element #1=w273:u16, element #2=w272:u16, element #3=w271:u16, element #4=w270:u16, element #5=w269:u16, element #6=w268:u16)  [unwired: 6 in]
            n115 = Boolean Array To Number(Boolean array=w279) -> (number=w278:u32)
            n116 = local read "READ SINUS PENTA"() -> (w283:T3)
            n117 = Bundle By Name(cluster=w283, "Menù ingressi digitali (M031-M036).Morsett comando da seriale"=w278, "Menù rampe (P009-P033).Tempo di acc rampa di vel 1"=w276, "Menù rampe (P009-P033).Tempo di dec rampa di vel 1"=w275, "Menù controllo motore(C008-C128).Freq nominale del motore Mot1"=w273, "Menù controllo motore(C008-C128).RPM nominali del motore Mot1"=w272, "Menù controllo motore(C008-C128).Potenza nominale del motore Mot1"=w271, "Menù controllo motore(C008-C128).Corrente nominale del motore Mot1"=w270, "Menù controllo motore(C008-C128).Tensione nominale del motore mot1"=w269, "Menù controllo motore(C008-C128).Velocità massima motore"=w268) -> (w282:T3)
          }
        }
        n118 = Bundle By Name(cluster=w122, "Comunicazione"=w120) -> (w121:T3)
        n119 = feedback-in #1(w118) -> ()
        n120 = feedback #1(errorcluster {"status"=FALSE, "code"=0, "source"=""} ("err in")) -> (w117:errorcluster)
        n121 = Bundle By Name(cluster=T4 {"Array of elements"=[], "Single element"={"String"="READ SINUS PENTA", "variant"=variant}, "enque at\nopposite end (F)"=FALSE, "no replications (F)"=FALSE} ("Enqueue cluster"), "Single element.variant"=w121) -> (w126:T4)
        n122 = case shown="Error" w117 {
          tunnel: w119 -> [w286 w289]
          frame No Error {
            n123 = Enqueue Element(queue=w286, element=cluster{"String":string, "variant":variant} {"String"="READ", "variant"=variant}) -> ()  [unwired: 2 in, 3 out]
          }
          frame Error {
            n124 = Flush Queue(queue=w289) -> (queue out=w288:refnum<queue>)  [unwired: 1 in, 2 out]
            n125 = Enqueue Element(queue=w288, element=cluster{"String":string, "variant":variant} {"String"="INITIALIZE", "variant"=variant}) -> ()  [unwired: 2 in, 3 out]
          }
        }
        n126 = call <userlib>:"SMQ_MANAGER.vi"("Function"=enum16{"INITIALIZE", "ENQUEUE", "STOP ALL"}."ENQUEUE", "Queue name"="DATA_Q", "Enqueue cluster"=w126) -> ()  [unwired: 8 in, 1 out]
      }
      frame "IDLE" {
        n127 = case shown="False" w298 {
          tunnel: w299 -> [w303 _]
          frame False {
            n128 = call-dynamic "Close.vi"("Modbus master in"=w303) -> ("error out"=w302:errorcluster)  [unwired: 10 in]
            n129 = call <vilib>:"Clear Errors.vi"("error in (no error)"=w302) -> ()  [unwired: 5 in, 2 out]
          }
          frame True {
          }
        }
        n130 = Flush Queue(queue=w300) -> ()  [unwired: 1 in, 3 out]
        n131 = local read "READ SINUS PENTA"() -> (w293:T3)
        n132 = Bundle By Name(cluster=w293, "Comunicazione"=FALSE) -> (w292:T3)
        n133 = Bundle By Name(cluster=T4 {"Array of elements"=[], "Single element"={"String"="READ SINUS PENTA", "variant"=variant}, "enque at\nopposite end (F)"=FALSE, "no replications (F)"=FALSE} ("Enqueue cluster"), "Single element.variant"=w292) -> (w297:T4)
        n134 = call <userlib>:"SMQ_MANAGER.vi"("Function"=enum16{"INITIALIZE", "ENQUEUE", "STOP ALL"}."ENQUEUE", "Queue name"="DATA_Q", "Enqueue cluster"=w297) -> ()  [unwired: 8 in, 1 out]
      }
      frame "WRITE REGISTER" {
        n135 = To Unsigned Word Integer(number="holding register values") -> (unsigned 16bit integer=w304:u16[])
        n136 = call-dynamic "Write Multiple Holding Registers.vi"("error in (no error)"=w306, "holding register values"=w304, "starting address"="starting address", "Modbus master in"=w310) -> ("error out"=w305:errorcluster, "Modbus master out"=w307:refnum<class "Modbus Master.lvclass">)  [unwired: 6 in]
      }
      frame "Senso rot" {
        n137 = Variant To Data(type=FALSE ("s"), Variant=w314) -> (data=w312:bool)  [unwired: 1 in, 1 out]
        n138 = case shown="False" w311 {
          tunnel: w318 -> [w326 w330]
          tunnel: w317 -> [w325 w329]
          tunnel: [w324 w329] -> w316
          tunnel: [w323 w330] -> w315
          tunnel: w312 -> [w319 _]
          frame False {
            n139 = Select(t=u16 1 ("senso rot"), s=w319, f=u16 0 ("senso rot")) -> (s? t:f=w320:u16)
            n140 = Build Array(w320) -> (w327:u16[])
            n141 = call-dynamic "Write Multiple Holding Registers.vi"("error in (no error)"=w325, "holding register values"=w327, "starting address"=u16 1014, "Modbus master in"=w326) -> ("error out"=w324:errorcluster, "Modbus master out"=w323:refnum<class "Modbus Master.lvclass">)  [unwired: 6 in]
          }
          frame True {
          }
        }
      }
      frame "Rif Velocità" {
        # "converto freq in rpm"
        n142 = local read "RPM nominali del motore Mot1"() -> (w331:u16)
        n143 = local read "Freq nominale del motore Mot1"() -> (w332:u16)
        n144 = Variant To Data(type=dbl[] [], Variant=w340) -> (data=w338:dbl[])  [unwired: 1 in, 1 out]
        n145 = Index Array(array=w338) -> (element #1=w337:dbl, element #2=w334:dbl)  [unwired: 2 in]
        n146 = Divide(x=w337, y=w332) -> (x/y=w336:dbl)
        n147 = Multiply(x=w336, y=w331) -> (x*y=w335:dbl)
        n148 = Build Array(w335, w334) -> (w333:dbl[])
        n149 = call-dynamic "Write Multiple Holding Registers.vi"("error in (no error)"=w343, "holding register values"=w333, "starting address"=u16 1412, "Modbus master in"=w345) -> ("error out"=w342:errorcluster, "Modbus master out"=w344:refnum<class "Modbus Master.lvclass">)  [unwired: 6 in]
      }
      frame "Rif Tensione" {
        n150 = Variant To Data(type=u16 0 ("Register"), Variant=w350) -> (data=w348:u16)  [unwired: 1 in, 1 out]
        n151 = Build Array(w348) -> (w346:u16[])
        n152 = call-dynamic "Write Multiple Holding Registers.vi"("error in (no error)"=w353, "holding register values"=w346, "starting address"=u16 1418, "Modbus master in"=w352) -> ("error out"=w349:errorcluster, "Modbus master out"=w351:refnum<class "Modbus Master.lvclass">)  [unwired: 6 in]
      }
      frame "Rif V&RPM" {
        # "converto freq in rpm"
        n153 = Variant To Data(type=cluster{"appended array":dbl[], "rif":u16} {"appended array"=[], "rif"=0}, Variant=w372) -> (data=w369:cluster{"appended array":dbl[], "rif":u16})  [unwired: 1 in, 1 out]
        n154 = Unbundle By Name(w369) -> ("appended array"=w357:dbl[], "rif"=w368:u16)
        n155 = Build Array(w368) -> (w371:u16[])
        n156 = call-dynamic "Write Multiple Holding Registers.vi"("error in (no error)"=w374, "holding register values"=w371, "starting address"=u16 1418, "Modbus master in"=w373) -> ("error out"=w359:errorcluster, "Modbus master out"=w361:refnum<class "Modbus Master.lvclass">)  [unwired: 6 in]
        n157 = local read "Freq nominale del motore Mot1"() -> (w356:u16)
        n158 = local read "RPM nominali del motore Mot1"() -> (w355:u16)
        n159 = Index Array(array=w357) -> (element #1=w366:dbl, element #2=w363:dbl)  [unwired: 2 in]
        n160 = Divide(x=w366, y=w356) -> (x/y=w365:dbl)
        n161 = Multiply(x=w365, y=w355) -> (x*y=w364:dbl)
        n162 = Build Array(w364, w363) -> (w362:dbl[])
        n163 = call-dynamic "Write Multiple Holding Registers.vi"("error in (no error)"=w359, "holding register values"=w362, "starting address"=u16 1412, "Modbus master in"=w361) -> ("error out"=w358:errorcluster, "Modbus master out"=w360:refnum<class "Modbus Master.lvclass">)  [unwired: 6 in]
      }
      frame "NoStart+Disable(0)" {
        w376 = FALSE ("Abilitato")
        w384 = u16 0  # Enable: MDI2
        n164 = Flush Queue(queue=w378) -> (queue out=w377:refnum<queue>)  [unwired: 1 in, 2 out]
        n165 = Build Array(w384) -> (w385:u16[])
        n166 = call-dynamic "Write Multiple Holding Registers.vi"("error in (no error)"=w383, "holding register values"=w385, "starting address"=u16 1406, "Modbus master in"=w381) -> ("error out"=w382:errorcluster, "Modbus master out"=w380:refnum<class "Modbus Master.lvclass">)  [unwired: 6 in]
        n167 = Enqueue Element(queue=w377, element=cluster{"String":string, "variant":variant} {"String"="READ", "variant"=variant}) -> ()  [unwired: 2 in, 3 out]
        n168 = local write "Abilitato"(w376) -> ()
        n169 = local write "in marcia"(w376) -> ()
      }
      frame "Start+Disable(1)" {
        w394 = u16 1  # Enable: MDI2
        n170 = Flush Queue(queue=w388) -> (queue out=w387:refnum<queue>)  [unwired: 1 in, 2 out]
        n171 = Build Array(w394) -> (w395:u16[])
        n172 = call-dynamic "Write Multiple Holding Registers.vi"("error in (no error)"=w390, "holding register values"=w395, "starting address"=u16 1406, "Modbus master in"=w392) -> ("error out"=w393:errorcluster, "Modbus master out"=w391:refnum<class "Modbus Master.lvclass">)  [unwired: 6 in]
        n173 = Enqueue Element(queue=w387, element=cluster{"String":string, "variant":variant} {"String"="READ", "variant"=variant}) -> ()  [unwired: 2 in, 3 out]
      }
      frame "Enable(2)" {
        w399 = u16 2  # Enable: MDI2
        n174 = Build Array(w399) -> (w407:u16[])
        n175 = Flush Queue(queue=w401) -> (queue out=w400:refnum<queue>)  [unwired: 1 in, 2 out]
        n176 = call-dynamic "Write Multiple Holding Registers.vi"("error in (no error)"=w404, "holding register values"=w407, "starting address"=u16 1406, "Modbus master in"=w406) -> ("error out"=w403:errorcluster, "Modbus master out"=w405:refnum<class "Modbus Master.lvclass">)  [unwired: 6 in]
        n177 = Enqueue Element(queue=w400, element=cluster{"String":string, "variant":variant} {"String"="READ", "variant"=variant}) -> ()  [unwired: 2 in, 3 out]
        n178 = local write "Abilitato"(TRUE ("Abilitato")) -> ()
        n179 = local write "in marcia"(FALSE ("in marcia")) -> ()
      }
      frame "Start+Enable(3)" {
        w409 = TRUE ("Abilitato")
        w410 = u16 3  # Enable+start: MDI2+MDI1
        n180 = Flush Queue(queue=w412) -> (queue out=w411:refnum<queue>)  [unwired: 1 in, 2 out]
        n181 = Enqueue Element(queue=w411, element=cluster{"String":string, "variant":variant} {"String"="READ", "variant"=variant}) -> ()  [unwired: 2 in, 3 out]
        n182 = Build Array(w410) -> (w418:u16[])
        n183 = call-dynamic "Write Multiple Holding Registers.vi"("error in (no error)"=w415, "holding register values"=w418, "starting address"=u16 1406, "Modbus master in"=w417) -> ("error out"=w414:errorcluster, "Modbus master out"=w416:refnum<class "Modbus Master.lvclass">)  [unwired: 6 in]
        n184 = local write "Abilitato"(w409) -> ()
        n185 = local write "in marcia"(w409) -> ()
      }
      frame "FreqCarrier2500" {
        n186 = local read "READ SINUS PENTA"() -> (w423:T3)
        n187 = Unbundle By Name(w423) -> ("ID"=w422:dbl)
        n188 = Not Equal?(x=w422, y=2.0) -> (x != y?=w420:bool)
        n189 = case shown="True" w420 {
          tunnel: w427 -> [w428 w433]
          tunnel: [w428 w432] -> w426
          tunnel: w425 -> [w429 w431]
          tunnel: [w429 w430] -> w424
          frame False {
          }
          frame True {
            n190 = flat-sequence {
              tunnel: w433 -> [w441]
              tunnel: w431 -> [w439]
              tunnel: [w440] -> w437
              tunnel: [w438] -> w436
              tunnel: w437 -> [w447]
              tunnel: w436 -> [w446]
              tunnel: [w447] -> w435
              tunnel: [w446] -> w434
              tunnel: [w448] -> w430
              tunnel: [w450] -> w432
              tunnel: w435 -> [w451]
              tunnel: w434 -> [w449]
              frame #0 {
                n191 = Build Array(u16 2500 ("Enable+start: MDI2+MDI1")) -> (w443:u16[])
                n192 = call-dynamic "Write Multiple Holding Registers.vi"("error in (no error)"=w441, "holding register values"=w443, "starting address"=u16 1002, "Modbus master in"=w439) -> ("error out"=w440:errorcluster, "Modbus master out"=w438:refnum<class "Modbus Master.lvclass">)  [unwired: 6 in]
              }
              frame #1 {
                n193 = Wait (ms)(milliseconds to wait=u32 250) -> ()  [unwired: 1 out]
              }
              frame #2 {
                n194 = Build Array(u16 2500 ("Enable+start: MDI2+MDI1")) -> (w453:u16[])
                n195 = call-dynamic "Write Multiple Holding Registers.vi"("error in (no error)"=w451, "holding register values"=w453, "starting address"=u16 1001, "Modbus master in"=w449) -> ("error out"=w450:errorcluster, "Modbus master out"=w448:refnum<class "Modbus Master.lvclass">)  [unwired: 6 in]
              }
            }
          }
        }
      }
      frame "FreqCarrier2200" {
        n196 = local read "READ SINUS PENTA"() -> (w458:T3)
        n197 = Unbundle By Name(w458) -> ("ID"=w457:dbl)
        n198 = Not Equal?(x=w457, y=2.0) -> (x != y?=w455:bool)
        n199 = case shown="True" w455 {
          tunnel: w462 -> [w464 w468]
          tunnel: [w464 w467] -> w461
          tunnel: w460 -> [w463 w466]
          tunnel: [w463 w465] -> w459
          frame False {
          }
          frame True {
            n200 = flat-sequence {
              tunnel: w466 -> [w476]
              tunnel: w468 -> [w474]
              tunnel: [w475] -> w472
              tunnel: [w473] -> w471
              tunnel: w472 -> [w482]
              tunnel: w471 -> [w481]
              tunnel: [w482] -> w470
              tunnel: [w481] -> w469
              tunnel: [w483] -> w467
              tunnel: [w485] -> w465
              tunnel: w470 -> [w486]
              tunnel: w469 -> [w484]
              frame #0 {
                n201 = Build Array(u16 2200 ("Enable+start: MDI2+MDI1")) -> (w478:u16[])
                n202 = call-dynamic "Write Multiple Holding Registers.vi"("error in (no error)"=w476, "holding register values"=w478, "starting address"=u16 1001, "Modbus master in"=w474) -> ("error out"=w475:errorcluster, "Modbus master out"=w473:refnum<class "Modbus Master.lvclass">)  [unwired: 6 in]
              }
              frame #1 {
                n203 = Wait (ms)(milliseconds to wait=u32 250) -> ()  [unwired: 1 out]
              }
              frame #2 {
                n204 = Build Array(u16 2200 ("Enable+start: MDI2+MDI1")) -> (w488:u16[])
                n205 = call-dynamic "Write Multiple Holding Registers.vi"("error in (no error)"=w486, "holding register values"=w488, "starting address"=u16 1002, "Modbus master in"=w484) -> ("error out"=w485:errorcluster, "Modbus master out"=w483:refnum<class "Modbus Master.lvclass">)  [unwired: 6 in]
              }
            }
          }
        }
      }
      frame "Set_Fmax" {
        # "1015: C015 Fnom motore\n1016: C016 Rpm motore"
        n206 = Variant To Data(type=u16 0 ("starting address"), Variant=w500) -> (data=w491:u16)  [unwired: 1 in, 1 out]
        n207 = Multiply(x=w491, y=u16 10) -> (x*y=w497:u16)
        n208 = Build Array(w497, w491) -> (w503:u16[])
        n209 = call-dynamic "Write Multiple Holding Registers.vi"("error in (no error)"=w502, "holding register values"=w503, "starting address"=u16 1015, "Modbus master in"=w501) -> ("error out"=w496:errorcluster, "Modbus master out"=w494:refnum<class "Modbus Master.lvclass">)  [unwired: 6 in]
        n210 = Build Array(w491) -> (w490:u16[])
        n211 = call-dynamic "Write Multiple Holding Registers.vi"("error in (no error)"=w496, "holding register values"=w490, "starting address"=u16 1029, "Modbus master in"=w494) -> ("error out"=w495:errorcluster, "Modbus master out"=w493:refnum<class "Modbus Master.lvclass">)  [unwired: 6 in]
      }
      frame "Stop" {
      }
      frame "Reset" {
        w507 = u16 4  # Reset: MDI3
        n212 = Build Array(w507) -> (w508:u16[])
        n213 = call-dynamic "Write Multiple Holding Registers.vi"("error in (no error)"=w513, "holding register values"=w508, "starting address"=u16 1406, "Modbus master in"=w512) -> ("error out"=w510:errorcluster, "Modbus master out"=w511:refnum<class "Modbus Master.lvclass">)  [unwired: 6 in]
      }
      frame "Imposta rampa" {
        n214 = Variant To Data(type=0.0, Variant=w522) -> (data=w514:dbl)  [unwired: 1 in, 1 out]
        n215 = global write "Global dati targa SINUSPENTA.vi" "Tempo rampa SINUS inviato"(TRUE ("Tempo rampa SINUS inviato")) -> ()
        n216 = Bundle By Name(cluster=T5 {"Trampa[s] acc"=0.0, "Trampa[s] dec"=0.0}, "Trampa[s] acc"=w514, "Trampa[s] dec"=w514) -> (w517:T5)
        n217 = Unbundle By Name(w517) -> ("Trampa[s] acc"=w520:dbl, "Trampa[s] dec"=w519:dbl)
        "data" <- w520
        "data 2" <- w519
        n218 = global write "Global dati targa SINUSPENTA.vi" "T rampa Intesys"(w514) -> ()
        n219 = case shown="False" w521 {
          tunnel: w526 -> [w535 w538]
          tunnel: w525 -> [w534 w537]
          tunnel: [w533 w538] -> w524
          tunnel: [w532 w537] -> w523
          tunnel: w520 -> [w529 _]
          tunnel: w519 -> [w527 _]
          frame False {
            n220 = Multiply(x=w529, y=1.0) -> (x*y=w528:dbl)
            n221 = Build Array(w528, w527) -> (w530:dbl[])
            n222 = call-dynamic "Write Multiple Holding Registers.vi"("error in (no error)"=w534, "holding register values"=w530, "starting address"=u16 609, "Modbus master in"=w535) -> ("error out"=w532:errorcluster, "Modbus master out"=w533:refnum<class "Modbus Master.lvclass">)  [unwired: 6 in]
          }
          frame True {
          }
        }
      }
      frame "Modalità stop" {
        # "0 deceleration ramp\n1 Free wheel"
        n223 = Variant To Data(type=i16 0, Variant=w543) -> (data=w539:i16)  [unwired: 1 in, 1 out]
        n224 = global write "Global dati targa SINUSPENTA.vi" "Tempo rampa SINUS inviato"(TRUE ("Tempo rampa SINUS inviato")) -> ()
        n225 = case shown="False" w542 {
          tunnel: w547 -> [w553 w556]
          tunnel: w546 -> [w552 w555]
          tunnel: [w551 w556] -> w545
          tunnel: [w550 w555] -> w544
          tunnel: w539 -> [w548 _]
          frame False {
            n226 = Build Array(w548) -> (w549:i16[])
            n227 = call-dynamic "Write Multiple Holding Registers.vi"("error in (no error)"=w552, "holding register values"=w549, "starting address"=u16 1185, "Modbus master in"=w553) -> ("error out"=w550:errorcluster, "Modbus master out"=w551:refnum<class "Modbus Master.lvclass">)  [unwired: 6 in]
          }
          frame True {
          }
        }
      }
      frame "Set dati targa motore" {
        w575 = u16 10 ("y")
        n228 = Variant To Data(type=T1 {"Freq nominale del motore Mot1"=0.0, "RPM nominali del motore Mot1"=0, "Potenza nominale del motore Mot1"=0.0, "Corrente nominale del motore Mot1"=0.0, "Tensione nominale del motore mot1"=0.0, "Rpm max"=0, "Modalità stop"=0} ("DATI TARGA sinus penta"), Variant=w583) -> (data=w561:T1)  [unwired: 1 in, 1 out]
        "DATI TARGA sinus penta" <- w561
        n229 = Unbundle By Name(w561) -> ("Freq nominale del motore Mot1"=w582:dbl, "RPM nominali del motore Mot1"=w574:i16, "Potenza nominale del motore Mot1"=w581:dbl, "Corrente nominale del motore Mot1"=w580:dbl, "Tensione nominale del motore mot1"=w579:dbl, "Rpm max"=w570:u16, "Modalità stop"=w557:u16)
        "RPM nominali del motore Mot1" <- w574
        "Freq nominale del motore Mot1" <- w582
        n230 = global write "Global dati targa SINUSPENTA.vi" "DATI TARGA sinus penta"(w561) -> ()
        n231 = Multiply(x=w582, y=w575) -> (x*y=w578:dbl)
        n232 = Multiply(x=w581, y=w575) -> (x*y=w563:dbl)
        n233 = Multiply(x=w580, y=w575) -> (x*y=w565:dbl)
        n234 = Multiply(x=w579, y=w575) -> (x*y=w567:dbl)
        n235 = global write "Global dati targa SINUSPENTA.vi" "Dati targa Sinus Inviati"(TRUE ("Tempo rampa SINUS inviato")) -> ()
        n236 = To Unsigned Word Integer(number=w578) -> (unsigned 16bit integer=w568:u16)
        n237 = To Unsigned Word Integer(number=w567) -> (unsigned 16bit integer=w566:u16)
        n238 = To Unsigned Word Integer(number=w563) -> (unsigned 16bit integer=w562:u16)
        n239 = To Unsigned Word Integer(number=w565) -> (unsigned 16bit integer=w564:u16)
        n240 = Build Array(w568, w574, w562, w564, w566) -> (w571:u16[])
        n241 = case shown="False" w572 {
          tunnel: w571 -> [w598 _]
          tunnel: w577 -> [w597 w601]
          tunnel: w576 -> [w596 w600]
          tunnel: [w586 w601] -> w558
          tunnel: [w584 w600] -> w559
          tunnel: w570 -> [w591 _]
          tunnel: w557 -> [w589 _]
          frame False {
            # "0 deceleration ramp\n1 Free wheel"
            n242 = call-dynamic "Write Multiple Holding Registers.vi"("error in (no error)"=w596, "holding register values"=w598, "starting address"=u16 1015, "Modbus master in"=w597) -> ("error out"=w593:errorcluster, "Modbus master out"=w594:refnum<class "Modbus Master.lvclass">)  [unwired: 6 in]
            n243 = Build Array(w591) -> (w592:u16[])
            n244 = call-dynamic "Write Multiple Holding Registers.vi"("error in (no error)"=w593, "holding register values"=w592, "starting address"=u16 1029, "Modbus master in"=w594) -> ("error out"=w585:errorcluster, "Modbus master out"=w587:refnum<class "Modbus Master.lvclass">)  [unwired: 6 in]
            n245 = Build Array(w589) -> (w590:u16[])
            n246 = call-dynamic "Write Multiple Holding Registers.vi"("error in (no error)"=w585, "holding register values"=w590, "starting address"=u16 1185, "Modbus master in"=w587) -> ("error out"=w584:errorcluster, "Modbus master out"=w586:refnum<class "Modbus Master.lvclass">)  [unwired: 6 in]
          }
          frame True {
          }
        }
        n247 = Build Array (concatenate)(w571, w570) -> (→"appended array":u16[])
      }
      frame "Exit" {
        n248 = property on="stop" class="Bool (strict)"("Val(Sgnl)"=TRUE ("Value (Signaling)")) -> ()  [unwired: 2 in, 2 out]
      }
    }
    "t" <- w57
    n249 = global write "Global dati targa SINUSPENTA.vi" "Errore Sinus"(w57) -> ()
    "Numeric" <- w71
  }
  n250 = while {
    tunnel: w43 -> [w608]
    tunnel: [w606] -> w31
    stop <- w607 stop-if-true
    # "PROCESSI A EVENTI"
    n251 = event shown="[4] \"set modalità stop\": Value Change" {
      selector: _ -> [_ _ _ _ _ _ _ _]
      dyn-events: [_ _ _ _ _ _ _ _] -> w606
      timeout: _ -> [_ _ _ _ _ _ _ _]
      tunnel: w608 -> [w610 w611 w613 w618 w622 w624 w627 w629]
      tunnel: [_ _ _ _ _ _ _ TRUE] -> w607
      event "write register": Value Change {
        n252 = event-data() -> ()  [unwired: 1 in, 2 out]
        n253 = Enqueue Element(queue=w610, element=cluster{"String":string, "variant":variant} {"String"="WRITE REGISTER", "variant"=variant}) -> ()  [unwired: 2 in, 3 out]
      }
      event "disconnetti": Value Change {
        n254 = event-data() -> ()  [unwired: 1 in, 2 out]
        n255 = Enqueue Element(queue=w611, element=cluster{"String":string, "variant":variant} {"String"="IDLE", "variant"=variant}) -> ()  [unwired: 2 in, 3 out]
      }
      event "connetti": Value Change {
        n256 = event-data() -> ()  [unwired: 1 in, 2 out]
        n257 = Enqueue Element(queue=w613, element=cluster{"String":string, "variant":variant} {"String"="INITIALIZE", "variant"=variant}) -> ()  [unwired: 2 in, 3 out]
      }
      event "set rampa": Value Change {
        n258 = event-data() -> ()  [unwired: 1 in, 2 out]
        n259 = Bundle By Name(cluster=cluster{"String":string, "variant":variant} {"String"="Imposta rampa", "variant"=variant} ("element"), "variant"="rampa") -> (w615:cluster{"String":string, "variant":variant})
        n260 = Enqueue Element(queue=w618, element=w615) -> ()  [unwired: 2 in, 3 out]
      }
      event "set modalità stop": Value Change {
        n261 = event-data() -> ()  [unwired: 1 in, 2 out]
        n262 = Bundle By Name(cluster=cluster{"String":string, "variant":variant} {"String"="Modalità stop", "variant"=variant} ("element"), "variant"="modalità stop") -> (w620:cluster{"String":string, "variant":variant})
        n263 = Enqueue Element(queue=w622, element=w620) -> ()  [unwired: 2 in, 3 out]
      }
      event "set dati targa": Value Change {
        n264 = event-data() -> ()  [unwired: 1 in, 2 out]
        n265 = Bundle By Name(cluster=cluster{"String":string, "variant":variant} {"String"="Set dati targa motore", "variant"=variant} ("element"), "variant"="DATI TARGA sinus penta 2") -> (w625:cluster{"String":string, "variant":variant})
        n266 = Enqueue Element(queue=w624, element=w625) -> ()  [unwired: 2 in, 3 out]
      }
      event "START ABILITA": Value Change {
        n267 = event-data() -> ()  [unwired: 1 in, 2 out]
        n268 = Enqueue Element(queue=w627, element=cluster{"String":string, "variant":variant} {"String"="Start+Enable(3)", "variant"=variant}) -> ()  [unwired: 2 in, 3 out]
      }
      event "stop": Value Change {
        n269 = event-data() -> ()  [unwired: 1 in, 2 out]
        n270 = Enqueue Element(queue=w629, element=cluster{"String":string, "variant":variant} {"String"="Exit", "variant"=variant}) -> ()  [unwired: 2 in, 3 out]
      }
    }
  }
  n271 = disable-structure shown="Disabled" {
    disable-tunnel: w31 -> [w632 _]
    frame Disabled {
      n272 = Unregister For Events(event registration refnum=w632) -> ()  [unwired: 1 in, 1 out]
    }
    frame Enabled {
    }
  }
  n273 = call-dynamic "Close.vi"("error in (no error)"=w33, "Modbus master in"=w34) -> ("error out"=w30:errorcluster)  [unwired: 9 in]
  n274 = call <vilib>:"Clear Errors.vi"("error in (no error)"=w30) -> ()  [unwired: 5 in, 2 out]
